vi "Read A.vi"(8 "error in (no error)":errorcluster, 11 "Analyze Results q-Factor in":refnum<class "Analyze Results q-Factor.lvclass">) -> (0 "error out":errorcluster, 2 "A":dbl[unit], 3 "Analyze Results q-Factor out":refnum<class "Analyze Results q-Factor.lvclass">)   [LabVIEW 2014, in "Analyze Results q-Factor.lvclass"]
uses:
  Analyze Results q-Factor.lvclass
  Analyze Results q-Factor.lvclass/Analyze Results q-Factor.ctl
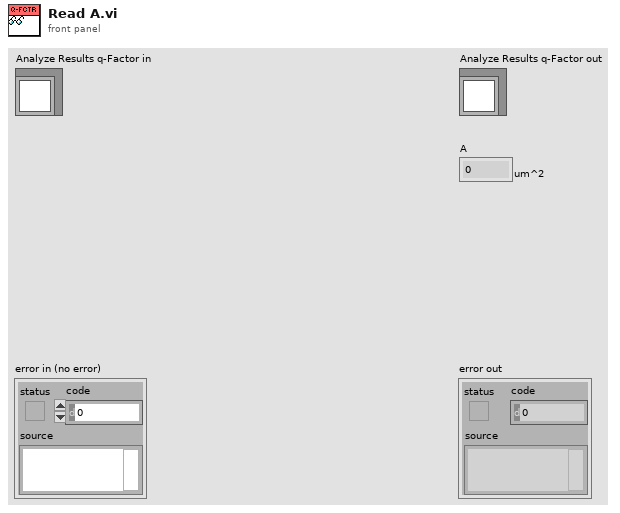
[diagram p1: front panel]
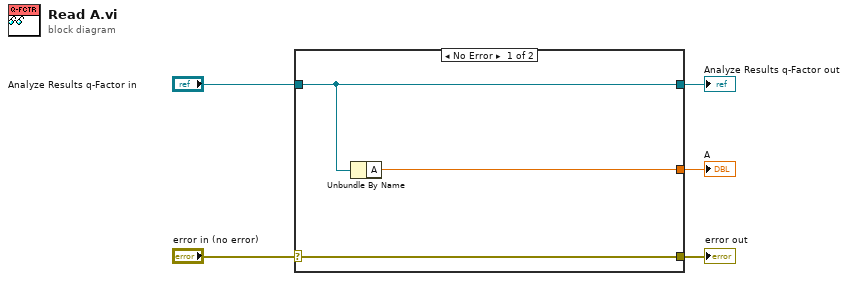
[diagram p0: block diagram]
diagram:
  n1 = case shown="No Error" "error in (no error)" {
    selector: "error in (no error)" -> [w8 w9]
    tunnel: [w8 w9] -> w4
    tunnel: [w7 w10] -> w2
    tunnel: "Analyze Results q-Factor in" -> [w7 w10]
    tunnel: [w6 _] -> w1
    frame No Error {
      n2 = Unbundle By Name(w7) -> ("A"=w6:dbl[unit])
    }
    frame Error {
    }
  }
  "error out" <- w4
  "Analyze Results q-Factor out" <- w2
  "A" <- w1
